vi "ellipsometry_220419.vi"() -> ()   [LabVIEW 2016]
uses:
  <vilib>/DAQmx/read.llb/DAQmx Read (Analog 1D DBL 1Chan NSamp).vi
  <vilib>/DAQmx/miscellaneous.llb/DAQmx Fill In Error Info.vi
panel:
  in  "?":enum32{"Gráfico"}(tab)
  out "?":cluster{"Y":dbl[], "Y":dbl[]}[](graph)=[{"Y"=[-4118.740370838965, -4287.913723170305, -4388.339578635604, -4445.957384510558, -4478.968400545135, -4430.379940252202, -4323.618309176339, -4199.467526974068, -4057.746052912791, -3899.317966754177, -3720.8720081576216, -3526.8237192438123, -3322.548224417388, -3104.161817602285, -2873.0919165381433, -2639.1427042346954, -2389.9909813235663, -2140.564686543254, -1881.9590478318137, -1624.4457888590766, -1367.5149473135568, -1107.9805939682005, -852.8381649863901, -591.654788435008, -330.0601398767841, -73.90728135941657, 185.33454633466167, 440.71743672506403, 698.016323996301, 953.2882778127398, 1206.5142592948591, 1457.8825071274605, 1704.6708108736004, 1962.185562370657, 2211.685572034808, 2457.842221707656, 2702.186375607056, 2943.573945737625, 3179.621751408952, 3411.9977643412653, 3643.8155013985875, 3858.596918122725, 4057.3951508943774, 4222.622419037125, 4353.076063627242, 4430.459463366088, 4475.65387782656, 4502.368449790882, 4517.767110991889, 4526.697914328664, 4531.890383619428, 4534.918840300799, 4536.827111619094, 4537.957802712025, 4538.700762058131, 4465.1933599331205, 4354.517492278845, 4226.984981778322, 4081.224105793564, 3917.6950482578795, 3736.72430132162, 3542.91095332093, 3333.572635169305, 3112.6414777688838, 2880.1530543014924, 2639.6207484627803, 2393.6793067215463, 2142.5740752883944, 1882.531978466757, 1631.6162264966895, 1364.7121502631694, 1105.4463526875065, 846.2080772288648, 588.2051621264471, 324.97305351691114, 66.10450927654243, -189.63173210680674, -442.84271030646255, -703.6869592985921, -959.9322377943728, -1213.6166923261712, -1465.7562171031884, -1716.3869314420667, -1970.5798522734574, -2218.5735637809034, -2466.041183335755, -2709.295684585094, -2952.4632875834777, -3189.348851665085, -3421.453399874245, -3647.370310619581, -3861.6142066812804, -4058.72231444826, -4221.698824049275, -4351.684736274453, -4427.271265180953, -4472.304290077205, -4498.18340402792, -4513.080136642858, -4521.493908276723], "Y"=[-0.35702017435232003, -0.3196664671654219, -0.2988918387180694, -0.2767306794728697, -0.27246202307904444, -0.2823279282360742, -0.30330877540376333, -0.33345647348374596, -0.36066571856334284, -0.40660422136729485, -0.4607215633195107, -0.51084043751975, -0.5588477227912256, -0.6173843332339882, -0.6682010975784028, -0.717315589046044, -0.7679279001801014, -0.823366608178037, -0.8817696978549058, -0.9481368517592543, -1.0111550137128211, -1.0714703063038848, -1.123900041959692, -1.181840210236752, -1.2497534755033128, -1.3087135132150371, -1.3632084964835636, -1.4194145893068417, -1.476693340851384, -1.5428380202496603, -1.5999600578397801, -1.6566289900128817, -1.7169154165993932, -1.77864773195038, -1.8586058361534845, -1.8835802982932017, -1.9477150008721886, -2.004737717976928, -2.061839177948201, -2.104300102557802, -2.1613774704687203, -2.217671978533254, -2.2721824259839596, -2.2990211552029782, -2.3313332706683223, -2.3437164076065464, -2.356597586355243, -2.3656267008583702, -2.373465633907601, -2.3753857544441312, -2.382616166342117, -2.3824635495241364, -2.3771881395640597, -2.374203169617891, -2.375398754725851, -2.3591135909802428, -2.33332022526568, -2.3047897213663835, -2.271787929241284, -2.2343290468791457, -2.1931572722204287, -2.146866774435176, -2.092544360315884, -2.040047343056865, -1.9870229563454114, -1.9302638062797193, -1.874592802041605, -1.8208118172928804, -1.7612862784386931, -1.7031621303079167, -1.637777965480187, -1.5750013266759508, -1.517862317916895, -1.4619115843447974, -1.4009629982000662, -1.3414087117465927, -1.2782741572178349, -1.2177991727923272, -1.1613451727044166, -1.111839854320927, -1.0566195838240129, -1.003179977833215, -0.9474560324783743, -0.8809155104853901, -0.8242345195400649, -0.7686194412819256, -0.7182919980464425, -0.6632055647077009, -0.60913781746325, -0.5522420570605447, -0.49787439784466647, -0.4475600451918731, -0.39938361085188695, -0.3673666817498665, -0.3317141507076667, -0.312933486150933, -0.30069287278338636, -0.29873735973233706, -0.29491402097747704, -0.28693269738594435]}]
  out "Fase\n Lock-In":dbl=-167.77608223214415
  out "DC Lock-In\n(V)":dbl=8.895511627197266
  out "AC Lock-In\n(mV)":dbl=-2.5524131458197425
  out "Valor do campo\n    magnético \n       (Gauss)":dbl=-4521.493908276723 format="%#.1p"
  in  "?":enum32{"Dados de Entrada"}(tab)
  in  "Pasta em que será salvo":path=path "E:/paniago/teste"
  in  "Nome do arquivo":string="teste_1"
  in  "Lock-In":cluster{"Ganho":u16, "Filtro TC":u16, "Ref":u16}={"Ganho"=2, "Filtro TC"=4, "Ref"=1} {"Ganho" items=["AC Gain 0 dB", "AC Gain 3 dB", "AC Gain 6 dB", "AC Gain 9 dB", "AC Gain 12 dB", "AC Gain 15 dB"]; "Ref" items=["Ref 1f", "Ref 2f"]; "Filtro TC" items=["TC 4ms", "TC 10ms", "TC 18ms", "TC 32ms", "TC 64ms", "TC 132ms", "TC 260ms", "TC 516ms"]}
  in  "Fase Lock-In\n    (Graus)":dbl
  in  "Pontos por \n  Segundo":u8=200
  in  "Campo de Saturação\n (Gauss)":dbl=200.0
  in  "Escala do Gaussimetro \n(Gauss)":u32(knob)=100 scale=100.0..10000.0
  in  "?":enum32{"Condições iniciais do motor de passo"}(tab)
  in  "Posição Inicial \n      (Graus)":dbl
  in  "Posição Final \n     (Graus)":dbl
  in  "?":bool
  in  "Enable \nMOTOR 1":bool=TRUE
  # "Sentido"
  # "Esquerda"
  # "Direita"
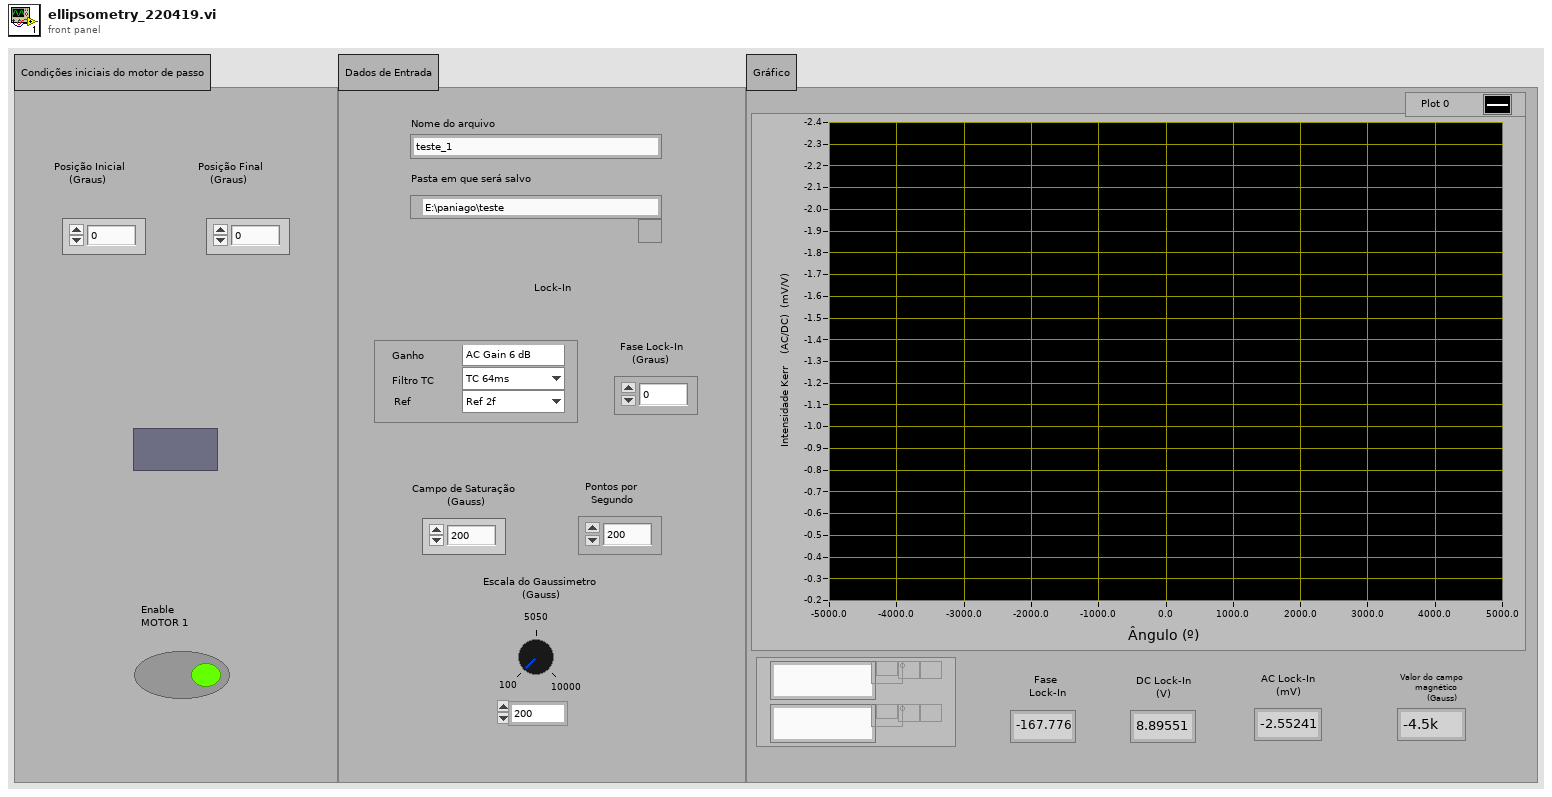
[diagram p1: front panel]
types:
  T1 = enum16{"open", "open or create", "create or replace", "create", "open (read only)"}
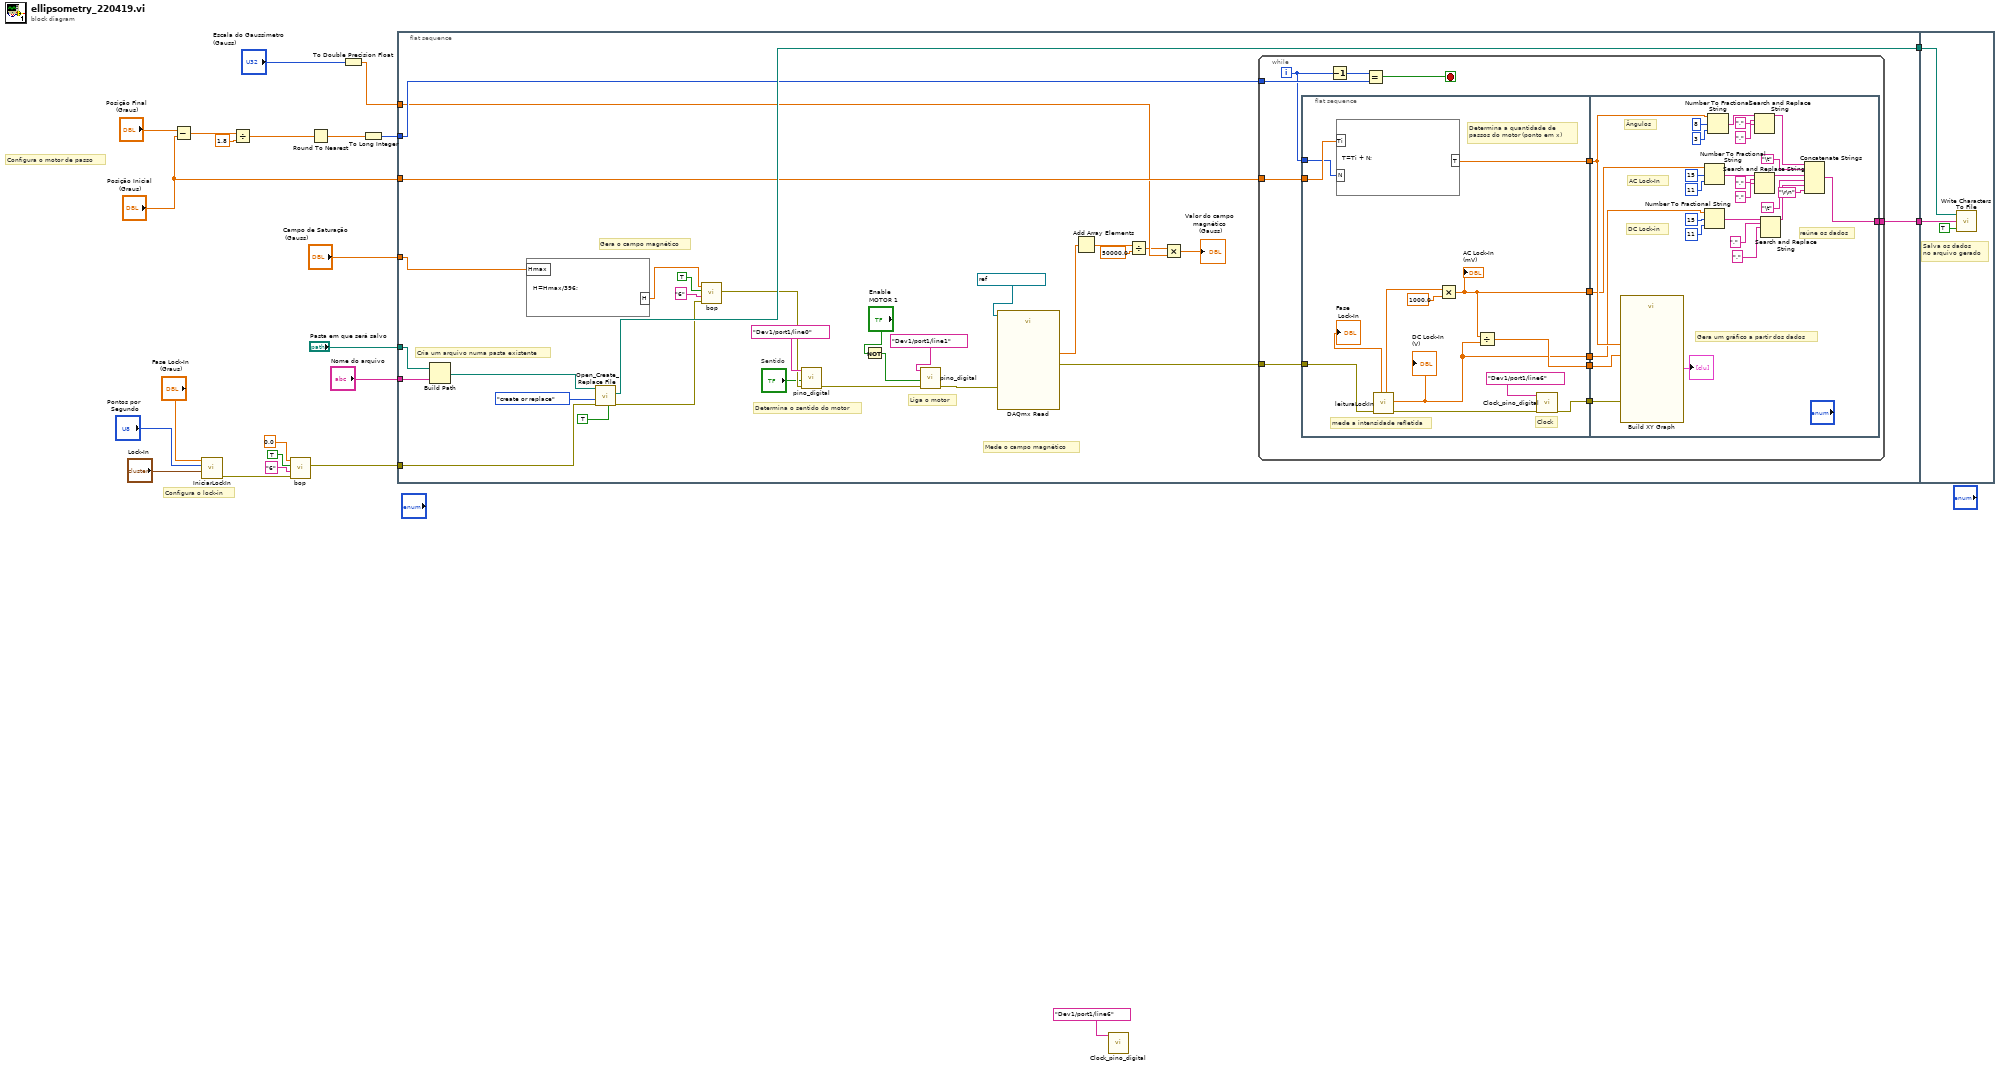
[diagram p0: block diagram]
diagram:
  # "Configura o lock-in"
  # "Configura o motor de passo"
  n1 = Subtract(x="Posição Final \n     (Graus)", y="Posição Inicial \n      (Graus)") -> (x-y=w22:dbl)
  n2 = call "IniciarLockIn.vi"("UserSelect"="Lock-In", "Points/sec"="Pontos por \n  Segundo", "Angle(deg)"="Fase Lock-In\n    (Graus)") -> ("error out"=w11:errorcluster)  [unwired: 6 in, 2 out]
  n3 = Divide(x=w22, y=1.8) -> (x/y=w21:dbl)
  n4 = call "bop.vi"("error in (no error)"=w11, "Endereço da Fonte"="6", "Boolean"=TRUE, "input 1"=0.0 ("Corrente")) -> ("error out"=w6:errorcluster)  [unwired: 4 in, 1 out]
  n5 = Round To Nearest(number=w21) -> (nearest integer value=w23:dbl)
  n6 = To Double Precision Float(number="Escala do Gaussimetro \n(Gauss)") -> (double precision float=w5:dbl)
  n7 = To Long Integer(number=w23) -> (32bit integer=w19:i32)
  n8 = flat-sequence {
    tunnel: w19 -> [w31]
    tunnel: "Campo de Saturação\n (Gauss)" -> [w48]
    tunnel: "Nome do arquivo" -> [w54]
    tunnel: "Pasta em que será salvo" -> [w53]
    tunnel: [w49] -> w14
    tunnel: "Posição Inicial \n      (Graus)" -> [w34]
    tunnel: w6 -> [w32]
    tunnel: w5 -> [w27]
    tunnel: [w24] -> w3
    tunnel: w14 -> [w109]
    tunnel: w3 -> [w108]
    frame #0 {
      # "Cria um arquivo numa pasta existente"
      # "Gera o campo magnético"
      # "Mede o campo magnético"
      # "Liga o motor"
      # "Determina o sentido do motor"
      # "Sentido"
      n9 = Build Path(base path=w53, name or relative path=w54) -> (appended path=w50:path)
      n10 = formula code="H=Hmax/396;"("Hmax"=w48) -> ("H"=w37:dbl)
      n11 = call <vilib>:"Open_Create_Replace File.vi"("advisory dialog? (display:T)"=TRUE, "error in (no error)"=w32, "function (open:0)"=T1."create or replace", "file path"=w50) -> ("error out"=w36:errorcluster, "new file path"=w49:path)  [unwired: 4 in, 2 out]
      n12 = call "bop.vi"("error in (no error)"=w36, "Endereço da Fonte"="6", "Boolean"=TRUE, "input 1"=w37) -> ("error out"=w42:errorcluster)  [unwired: 4 in, 1 out]
      n13 = call "pino_digital.vi"("error in"=w42, "data"="?", "lines"=tag "Dev1/port1/line0") -> ("error out"=w43:errorcluster)  [unwired: 8 in]
      n14 = Not(x="Enable \nMOTOR 1") -> (.not. x?=w38:bool)
      n15 = call "pino_digital.vi"("error in"=w43, "data"=w38, "lines"=tag "Dev1/port1/line1") -> ("error out"=w41:errorcluster)  [unwired: 8 in]
      n16 = call-poly <vilib>:"DAQmx Read.vi"("task/channels in"=refnum<k21> "ai0_SondaHall", "error in"=w41) -> ("data"=w28:dbl[], "error out"=w33:errorcluster)  [unwired: 11 in, 1 out]
      n17 = Add Array Elements(numeric array=w28) -> (sum=w30:dbl)
      n18 = Divide(x=w30, y=50000.0) -> (x/y=w26:dbl)
      n19 = Multiply(x=w26, y=w27) -> (x*y=→"Valor do campo\n    magnético \n       (Gauss)":dbl)
      n20 = while {
        tunnel: w34 -> [w66]
        tunnel: w33 -> [w64]
        tunnel: w31 -> [w62]
        tunnel: [w55] -> w24
        i -> [w61]
        stop <- w63 stop-if-true
        n21 = flat-sequence {
          tunnel: w66 -> [w78]
          tunnel: w61 -> [w75]
          tunnel: [w77] -> w65
          tunnel: w64 -> [w74]
          tunnel: [w72] -> w59
          tunnel: [w69] -> w58
          tunnel: [w68] -> w57
          tunnel: [w67] -> w56
          tunnel: w65 -> [w83]
          tunnel: w59 -> [w106]
          tunnel: w58 -> [w105]
          tunnel: w57 -> [w82]
          tunnel: w56 -> [w81]
          tunnel: [w80] -> w55
          frame #0 {
            # "Clock"
            # "mede a intensidade refletida"
            # "Determina a quantidade de\npassos do motor (ponto em x)"
            n22 = formula code="T=Ti + N;"("Ti"=w78, "N"=w75) -> ("T"=w77:dbl)
            n23 = call "leituraLockIn.vi"("error in (no error)"=w74) -> ("error out"=w73:errorcluster, "DC Volts"=w68:dbl, "X Volts RMS 2"=w70:dbl, "Fase"=→"Fase\n Lock-In":dbl)  [unwired: 5 in, 2 out]
            "DC Lock-In\n(V)" <- w68
            n24 = Multiply(x=w70, y=1000.0) -> (x*y=w67:dbl)
            "AC Lock-In\n(mV)" <- w67
            n25 = Divide(x=w67, y=w68) -> (x/y=w69:dbl)
            n26 = call "Clock_pino_digital.vi"("error in"=w73, "lines"=tag "Dev1/port1/line6") -> ("error out"=w72:errorcluster)  [unwired: 9 in]
          }
          frame #1 {
            # "DC Lock-in"
            # "AC Lock-In"
            # "Ângulos"
            # "Gera um gráfico a partir dos dados"
            # "reúne os dados"
            n27 = call "Build XY Graph"("error in (no error)"=w106, "Y Input"=w105, "X Input"=w83) -> ("XY Graph"=→"?":cluster{"Y":dbl[], "Y":dbl[]}[])  [unwired: 7 in, 1 out]
            n28 = Number To Fractional String(number=w81, width (-)=i16 15, precision (6)=i16 11) -> (F-format string=w97:string)  [unwired: 1 in]
            n29 = Number To Fractional String(number=w82, width (-)=i16 15, precision (6)=i16 11) -> (F-format string=w99:string)  [unwired: 1 in]
            n30 = Number To Fractional String(number=w83, width (-)=i16 8, precision (6)=i16 3) -> (F-format string=w88:string)  [unwired: 1 in]
            n31 = Search and Replace String(input string=w88, search string=",", replace string="." ("replace string (\"\")")) -> (result string=w87:string)  [unwired: 5 in, 3 out]
            n32 = Search and Replace String(input string=w97, search string=",", replace string="." ("replace string (\"\")")) -> (result string=w98:string)  [unwired: 5 in, 3 out]
            n33 = Search and Replace String(input string=w99, search string=",", replace string="." ("replace string (\"\")")) -> (result string=w100:string)  [unwired: 5 in, 3 out]
            n34 = Concatenate Strings(w87, "\t", w98, "\t", w100, "\r\n") -> (w80:string)
          }
        }
        n35 = Decrement(x=w61) -> (x-1=w60:i32)
        n36 = Equal?(x=w60, y=w62) -> (x = y?=w63:bool)
      }
    }
    frame #1 {
      # "Salva os dados \nno arquivo gerado"
      n37 = call <vilib>:"Write Characters To File.vi"("append to file? (new file:F)"=TRUE, "character string"=w108, "file path (dialog if empty)"=w109) -> ()  [unwired: 2 in, 1 out]
    }
  }
  n38 = call "Clock_pino_digital.vi"("lines"=tag "Dev1/port1/line6") -> ()  [unwired: 10 in, 1 out]
